vi "Principal.vi"() -> ()   [LabVIEW 2018]
panel:
  out "Time":string
  out "Date":string
  out "VIs ref":refnum<vi>[](array[refnum])
  in  "Reports":bool
  in  "Network":bool
  in  "Configuration":bool
  in  "Trends":bool
  in  "Overview":bool
  in  "Return 2":bool
  in  "Return":bool
  in  "Boton Tanque 4":bool
  out "Tank 4":dbl(slide)=80.0 scale=0.0..100.0 scale format="%#_g%%"
  out "Pressure 4":dbl=14.0 format="%#_g psi"
  out "Fuel Level 4":dbl=800.0 format="%#_g L"
  out "Temperature 4":dbl=60.0 format="%#_g °C"
  out "Percentage 4":dbl=80.0 format="%#_g %%"
  in  "Boton Tanque 3":bool
  out "Tank 3":dbl(slide)=60.0 scale=0.0..100.0 scale format="%#_g%%"
  out "Pressure 3":dbl=13.0 format="%#_g psi"
  out "Fuel Level 3":dbl=600.0 format="%#_g L"
  out "Temperature 3":dbl=45.0 format="%#_g °C"
  out "Percentage 3":dbl=60.0 format="%#_g %%"
  in  "Boton Tanque 2":bool
  out "Tank 2":dbl(slide)=40.0 scale=0.0..100.0 scale format="%#_g%%"
  out "Pressure 2":dbl=12.0 format="%#_g psi"
  out "Fuel Level 2":dbl=400.0 format="%#_g L"
  out "Temperature 2":dbl=30.0 format="%#_g °C"
  out "Percentage 2":dbl=40.0 format="%#_g %%"
  in  "Boton Tanque 1":bool
  out "Tank 1":dbl(slide)=20.0 scale=0.0..100.0 scale format="%#_g%%"
  out "Pressure":dbl=11.0 format="%#_g psi"
  out "Fuel Level":dbl=200.0 format="%#_g L"
  out "Temperature":dbl=15.0 format="%#_g °C"
  out "Percentage":dbl=20.0 format="%.0f %%"
  in  "stop":bool
  in  "SideTank4":bool
  in  "SideTank3":bool
  in  "SideTank2":bool
  in  "SideTank1":bool
  in  "Down Button":bool
  in  "Up Button":bool
  out "Multicolumn Listbox":i32(listbox)=5
  # "Fuel Tanks Gauging System - Tanks Courtyard \"Name\""
  # "View Tanks Details"
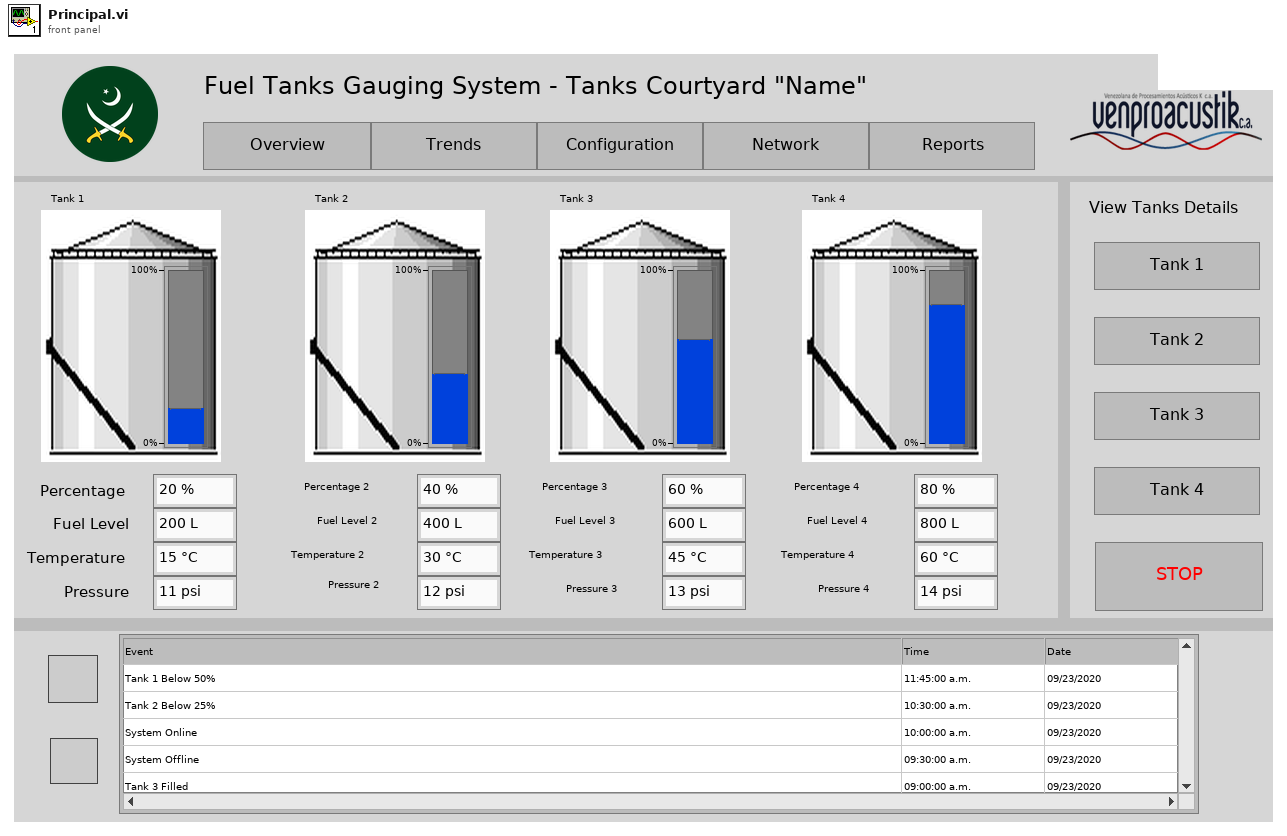
[diagram p1: front panel]
types:
  T1 = cluster{"Pressure":dbl, "Fuel Level":dbl, "Temperature":dbl, "Percentage":dbl}
  T2 = cluster{"Pressure 2":dbl, "Fuel Level 2":dbl, "Temperature 2":dbl, "Percentage 2":dbl}
  T3 = cluster{"Pressure 3":dbl, "Fuel Level 3":dbl, "Temperature 3":dbl, "Percentage 3":dbl}
  T4 = cluster{"Pressure 4":dbl, "Fuel Level 4":dbl, "Temperature 4":dbl, "Percentage 4":dbl}
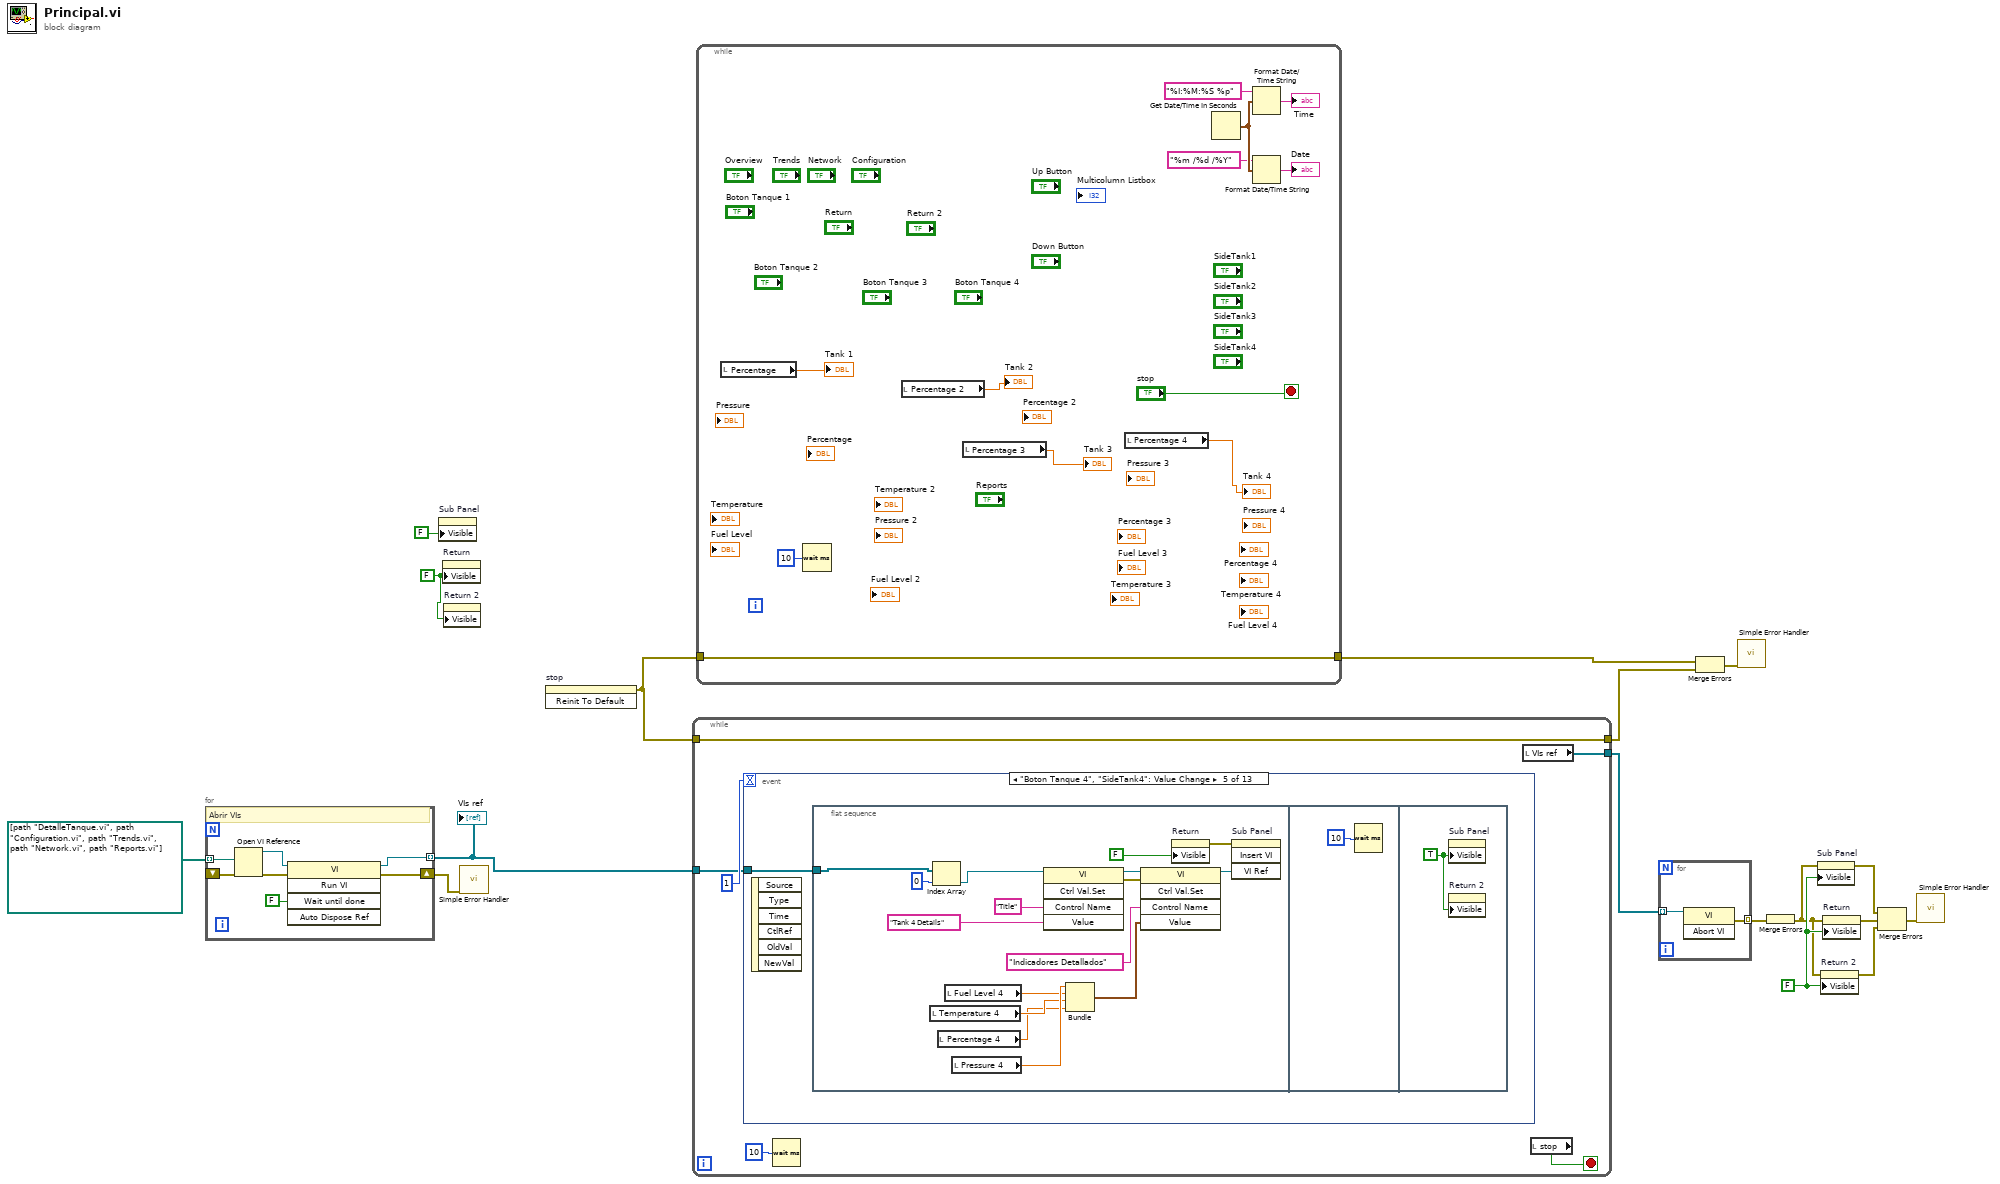
[diagram p0: block diagram]
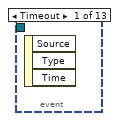
[diagram p2: hidden frame]
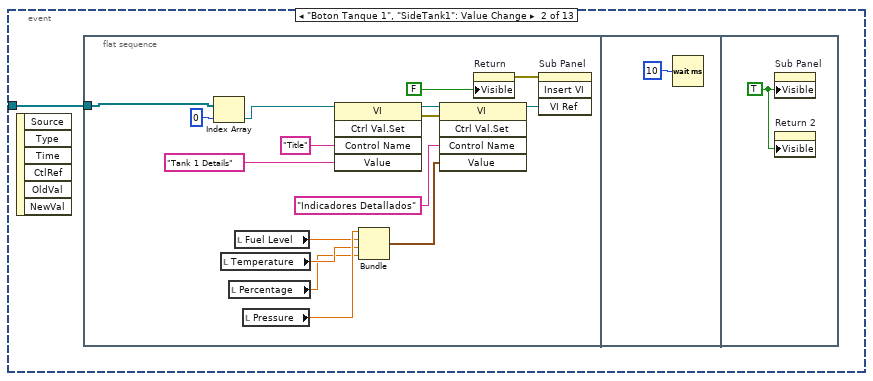
[diagram p3: hidden frame]
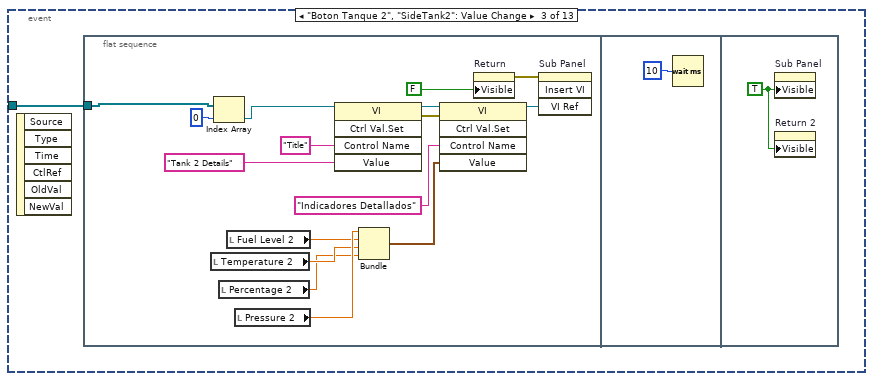
[diagram p4: hidden frame]
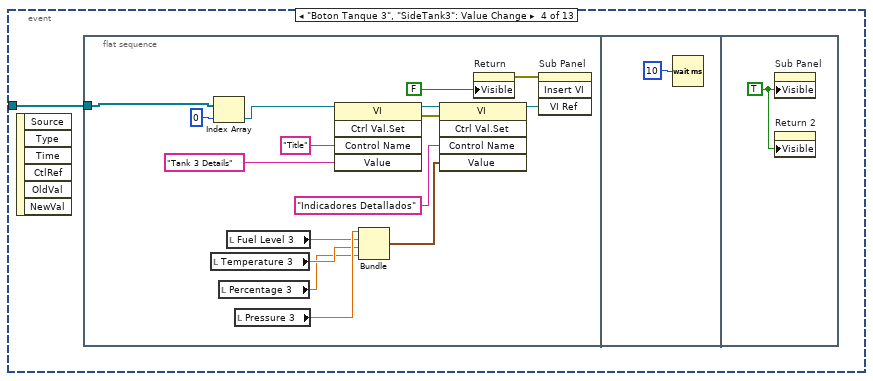
[diagram p5: hidden frame]
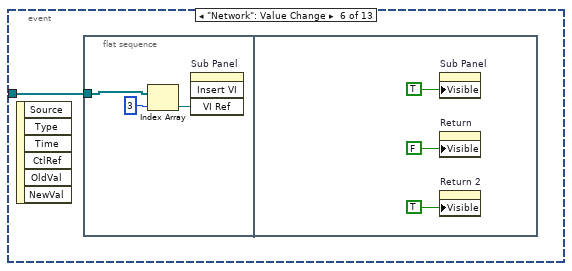
[diagram p6: hidden frame]
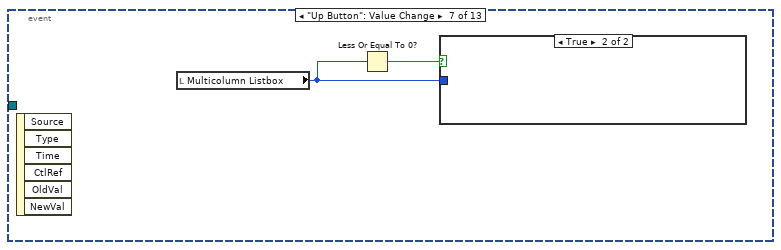
[diagram p7: hidden frame]
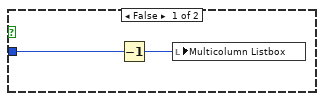
[diagram p8: hidden frame]
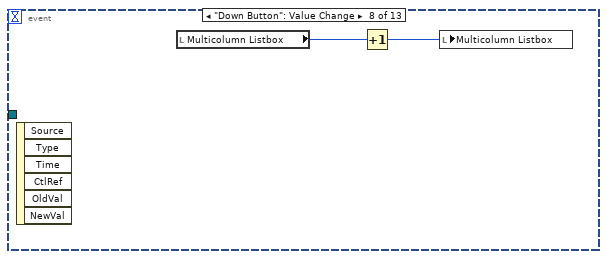
[diagram p9: hidden frame]
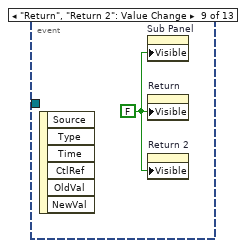
[diagram p10: hidden frame]
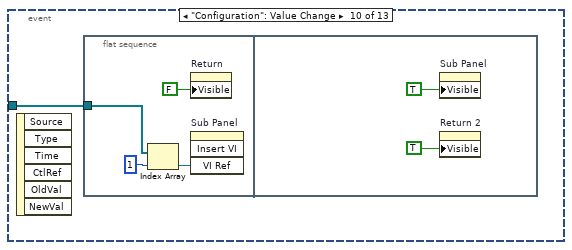
[diagram p11: hidden frame]
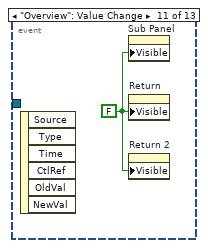
[diagram p12: hidden frame]
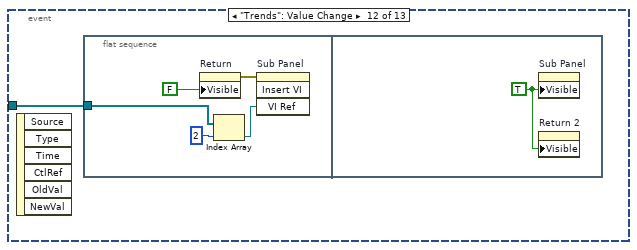
[diagram p13: hidden frame]
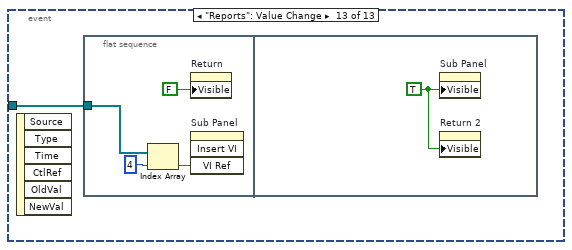
[diagram p14: hidden frame]
diagram:
  w7 = FALSE ("Visible")
  w8 = FALSE ("Visible")
  n1 = for {
    tunnel: path[] [path "DetalleTanque.vi", path "Configuration.vi", path "Trends.vi", path "Network.vi", path "Reports.vi"] -> [w24] mode=indexing
    shift-right: [w20] -> w12
    shift-left: _ -> [w19]
    tunnel: [w18] -> w1 mode=indexing
    # "Abrir VIs"
    n2 = Open VI Reference(vi path=w24, error in (no error)=w19) -> (vi reference=w22:refnum<vi>, error out=w21:errorcluster)  [unwired: 4 in]
    n3 = invoke class="VI" method="Run VI"(reference=w22, error in=w21, "Wait until done"=FALSE ("Wait Until Done")) -> (reference out=w18:refnum<vi>, error out=w20:errorcluster)  [unwired: 2 in, 3 out]
  }
  "VIs ref" <- w1
  n4 = property on="Sub Panel" class="SubPnl"("Visible"=FALSE) -> ()  [unwired: 2 in, 2 out]
  n5 = property on="Return" class="Bool"("Visible"=w8) -> ()  [unwired: 2 in, 2 out]
  n6 = property on="Return 2" class="Bool"("Visible"=w8) -> ()  [unwired: 2 in, 2 out]
  n7 = call <vilib>:"Simple Error Handler.vi"("error in (no error)"=w12) -> ()  [unwired: 4 in, 5 out]
  n8 = invoke on="stop" class="Bool (strict)" method="Reinit To Default"() -> (error out=w9:errorcluster)  [unwired: 3 in, 2 out]
  n9 = while {
    tunnel: w9 -> [w28]
    tunnel: [w28] -> w15
    tunnel: w1 -> [w27]
    tunnel: [w26] -> w11
    stop <- w29 stop-if-true
    n10 = event shown="[4] \"Boton Tanque 4\", \"SideTank4\": Value Change" {
      selector: _ -> [_ _ _ _ _ _ _ _ _ _ _ _ _]
      dyn-events: _ -> [_ _ _ _ _ _ _ _ _ _ _ _ _]
      timeout: 1 -> [_ _ _ _ _ _ _ _ _ _ _ _ _]
      tunnel: w27 -> [_ w31 w50 w69 w88 w107 _ _ _ w121 _ w129 w136]
      event Timeout {
        n11 = event-data() -> ()  [unwired: 1 in, 3 out]
      }
      event "Boton Tanque 1", "SideTank1": Value Change {
        n12 = event-data() -> ()  [unwired: 1 in, 6 out]
        n13 = flat-sequence {
          tunnel: w31 -> [w36]
          frame #0 {
            n14 = Index Array(array=w36, index=0) -> (element=w35:refnum<vi>)
            n15 = local read "Temperature"() -> (w41:dbl)
            n16 = local read "Percentage"() -> (w40:dbl)
            n17 = local read "Fuel Level"() -> (w42:dbl)
            n18 = local read "Pressure"() -> (w43:dbl)
            n19 = invoke class="VI" method="Ctrl Val.Set"(reference=w35, "Control Name"="Title", "Value"="Tank 1 Details" ("Control Name")) -> (reference out=w45:refnum<vi>, error out=w44:errorcluster)  [unwired: 2 in, 3 out]
            n20 = Bundle("Pressure"=w43, "Fuel Level"=w42, "Temperature"=w41, "Percentage"=w40) -> (w37:T1)  [unwired: 1 in]
            n21 = invoke class="VI" method="Ctrl Val.Set"(reference=w45, error in=w44, "Control Name"="Indicadores Detallados", "Value"=w37) -> (reference out=w38:refnum<vi>)  [unwired: 1 in, 4 out]
            n22 = property on="Return" class="Bool"("Visible"=FALSE) -> (error out=w32:errorcluster)  [unwired: 2 in, 1 out]
            n23 = invoke on="Sub Panel" class="SubPnl" method="Insert VI"(error in=w32, "VI Ref"=w38) -> ()  [unwired: 2 in, 4 out]
          }
          frame #1 {
            n24 = Wait (ms)(milliseconds to wait=u32 10) -> ()  [unwired: 1 out]
          }
          frame #2 {
            w49 = TRUE ("Visible")
            n25 = property on="Sub Panel" class="SubPnl"("Visible"=w49) -> ()  [unwired: 2 in, 2 out]
            n26 = property on="Return 2" class="Bool"("Visible"=w49) -> ()  [unwired: 2 in, 2 out]
          }
        }
      }
      event "Boton Tanque 2", "SideTank2": Value Change {
        n27 = event-data() -> ()  [unwired: 1 in, 6 out]
        n28 = flat-sequence {
          tunnel: w50 -> [w53]
          frame #0 {
            n29 = local read "Temperature 2"() -> (w60:dbl)
            n30 = Index Array(array=w53, index=0) -> (element=w54:refnum<vi>)
            n31 = local read "Percentage 2"() -> (w59:dbl)
            n32 = local read "Fuel Level 2"() -> (w61:dbl)
            n33 = local read "Pressure 2"() -> (w62:dbl)
            n34 = invoke class="VI" method="Ctrl Val.Set"(reference=w54, "Control Name"="Title", "Value"="Tank 2 Details" ("Control Name")) -> (reference out=w64:refnum<vi>, error out=w63:errorcluster)  [unwired: 2 in, 3 out]
            n35 = Bundle("Pressure 2"=w62, "Fuel Level 2"=w61, "Temperature 2"=w60, "Percentage 2"=w59) -> (w56:T2)  [unwired: 1 in]
            n36 = invoke class="VI" method="Ctrl Val.Set"(reference=w64, error in=w63, "Control Name"="Indicadores Detallados", "Value"=w56) -> (reference out=w57:refnum<vi>)  [unwired: 1 in, 4 out]
            n37 = property on="Return" class="Bool"("Visible"=FALSE) -> (error out=w51:errorcluster)  [unwired: 2 in, 1 out]
            n38 = invoke on="Sub Panel" class="SubPnl" method="Insert VI"(error in=w51, "VI Ref"=w57) -> ()  [unwired: 2 in, 4 out]
          }
          frame #1 {
            n39 = Wait (ms)(milliseconds to wait=u32 10) -> ()  [unwired: 1 out]
          }
          frame #2 {
            w68 = TRUE ("Visible")
            n40 = property on="Sub Panel" class="SubPnl"("Visible"=w68) -> ()  [unwired: 2 in, 2 out]
            n41 = property on="Return 2" class="Bool"("Visible"=w68) -> ()  [unwired: 2 in, 2 out]
          }
        }
      }
      event "Boton Tanque 3", "SideTank3": Value Change {
        n42 = event-data() -> ()  [unwired: 1 in, 6 out]
        n43 = flat-sequence {
          tunnel: w69 -> [w73]
          frame #0 {
            n44 = local read "Temperature 3"() -> (w79:dbl)
            n45 = Index Array(array=w73, index=0) -> (element=w72:refnum<vi>)
            n46 = local read "Percentage 3"() -> (w78:dbl)
            n47 = local read "Fuel Level 3"() -> (w80:dbl)
            n48 = local read "Pressure 3"() -> (w81:dbl)
            n49 = invoke class="VI" method="Ctrl Val.Set"(reference=w72, "Control Name"="Title", "Value"="Tank 3 Details" ("Control Name")) -> (reference out=w83:refnum<vi>, error out=w82:errorcluster)  [unwired: 2 in, 3 out]
            n50 = Bundle("Pressure 3"=w81, "Fuel Level 3"=w80, "Temperature 3"=w79, "Percentage 3"=w78) -> (w75:T3)  [unwired: 1 in]
            n51 = invoke class="VI" method="Ctrl Val.Set"(reference=w83, error in=w82, "Control Name"="Indicadores Detallados", "Value"=w75) -> (reference out=w76:refnum<vi>)  [unwired: 1 in, 4 out]
            n52 = property on="Return" class="Bool"("Visible"=FALSE) -> (error out=w71:errorcluster)  [unwired: 2 in, 1 out]
            n53 = invoke on="Sub Panel" class="SubPnl" method="Insert VI"(error in=w71, "VI Ref"=w76) -> ()  [unwired: 2 in, 4 out]
          }
          frame #1 {
            n54 = Wait (ms)(milliseconds to wait=u32 10) -> ()  [unwired: 1 out]
          }
          frame #2 {
            w87 = TRUE ("Visible")
            n55 = property on="Sub Panel" class="SubPnl"("Visible"=w87) -> ()  [unwired: 2 in, 2 out]
            n56 = property on="Return 2" class="Bool"("Visible"=w87) -> ()  [unwired: 2 in, 2 out]
          }
        }
      }
      event "Boton Tanque 4", "SideTank4": Value Change {
        n57 = event-data() -> ()  [unwired: 1 in, 6 out]
        n58 = flat-sequence {
          tunnel: w88 -> [w92]
          frame #0 {
            n59 = local read "Temperature 4"() -> (w98:dbl)
            n60 = Index Array(array=w92, index=0) -> (element=w91:refnum<vi>)
            n61 = local read "Percentage 4"() -> (w97:dbl)
            n62 = local read "Fuel Level 4"() -> (w99:dbl)
            n63 = local read "Pressure 4"() -> (w100:dbl)
            n64 = invoke class="VI" method="Ctrl Val.Set"(reference=w91, "Control Name"="Title", "Value"="Tank 4 Details" ("Control Name")) -> (reference out=w102:refnum<vi>, error out=w101:errorcluster)  [unwired: 2 in, 3 out]
            n65 = Bundle("Pressure 4"=w100, "Fuel Level 4"=w99, "Temperature 4"=w98, "Percentage 4"=w97) -> (w94:T4)  [unwired: 1 in]
            n66 = invoke class="VI" method="Ctrl Val.Set"(reference=w102, error in=w101, "Control Name"="Indicadores Detallados", "Value"=w94) -> (reference out=w95:refnum<vi>)  [unwired: 1 in, 4 out]
            n67 = property on="Return" class="Bool"("Visible"=FALSE) -> (error out=w89:errorcluster)  [unwired: 2 in, 1 out]
            n68 = invoke on="Sub Panel" class="SubPnl" method="Insert VI"(error in=w89, "VI Ref"=w95) -> ()  [unwired: 2 in, 4 out]
          }
          frame #1 {
            n69 = Wait (ms)(milliseconds to wait=u32 10) -> ()  [unwired: 1 out]
          }
          frame #2 {
            w106 = TRUE ("Visible")
            n70 = property on="Sub Panel" class="SubPnl"("Visible"=w106) -> ()  [unwired: 2 in, 2 out]
            n71 = property on="Return 2" class="Bool"("Visible"=w106) -> ()  [unwired: 2 in, 2 out]
          }
        }
      }
      event "Network": Value Change {
        n72 = event-data() -> ()  [unwired: 1 in, 6 out]
        n73 = flat-sequence {
          tunnel: w107 -> [w108]
          frame #0 {
            n74 = Index Array(array=w108, index=3) -> (element=w109:refnum<vi>)
            n75 = invoke on="Sub Panel" class="SubPnl" method="Insert VI"("VI Ref"=w109) -> ()  [unwired: 3 in, 4 out]
          }
          frame #1 {
            n76 = property on="Sub Panel" class="SubPnl"("Visible"=TRUE) -> ()  [unwired: 2 in, 2 out]
            n77 = property on="Return" class="Bool"("Visible"=FALSE) -> ()  [unwired: 2 in, 2 out]
            n78 = property on="Return 2" class="Bool"("Visible"=TRUE) -> ()  [unwired: 2 in, 2 out]
          }
        }
      }
      event "Up Button": Value Change {
        n79 = event-data() -> ()  [unwired: 1 in, 6 out]
        n80 = local read "Multicolumn Listbox"() -> (w114:i32)
        n81 = Less Or Equal To 0?(x=w114) -> (x <= 0?=w115:bool)
        n82 = case shown="True" w115 {
          tunnel: w114 -> [w116 _]
          frame False {
            n83 = Decrement(x=w116) -> (x-1=w117:i32)
            n84 = local write "Multicolumn Listbox"(w117) -> ()
          }
          frame True {
          }
        }
      }
      event "Down Button": Value Change {
        n85 = event-data() -> ()  [unwired: 1 in, 6 out]
        n86 = local read "Multicolumn Listbox"() -> (w119:i32)
        n87 = Increment(x=w119) -> (x+1=w118:i32)
        n88 = local write "Multicolumn Listbox"(w118) -> ()
      }
      event "Return", "Return 2": Value Change {
        w120 = FALSE ("Visible")
        n89 = event-data() -> ()  [unwired: 1 in, 6 out]
        n90 = property on="Sub Panel" class="SubPnl"("Visible"=w120) -> ()  [unwired: 2 in, 2 out]
        n91 = property on="Return" class="Bool"("Visible"=w120) -> ()  [unwired: 2 in, 2 out]
        n92 = property on="Return 2" class="Bool"("Visible"=w120) -> ()  [unwired: 2 in, 2 out]
      }
      event "Configuration": Value Change {
        n93 = event-data() -> ()  [unwired: 1 in, 6 out]
        n94 = flat-sequence {
          tunnel: w121 -> [w124]
          frame #0 {
            n95 = Index Array(array=w124, index=1) -> (element=w123:refnum<vi>)
            n96 = property on="Return" class="Bool"("Visible"=FALSE) -> ()  [unwired: 2 in, 2 out]
            n97 = invoke on="Sub Panel" class="SubPnl" method="Insert VI"("VI Ref"=w123) -> ()  [unwired: 3 in, 4 out]
          }
          frame #1 {
            n98 = property on="Sub Panel" class="SubPnl"("Visible"=TRUE) -> ()  [unwired: 2 in, 2 out]
            n99 = property on="Return 2" class="Bool"("Visible"=TRUE) -> ()  [unwired: 2 in, 2 out]
          }
        }
      }
      event "Overview": Value Change {
        w128 = FALSE ("Visible")
        n100 = event-data() -> ()  [unwired: 1 in, 6 out]
        n101 = property on="Sub Panel" class="SubPnl"("Visible"=w128) -> ()  [unwired: 2 in, 2 out]
        n102 = property on="Return" class="Bool"("Visible"=w128) -> ()  [unwired: 2 in, 2 out]
        n103 = property on="Return 2" class="Bool"("Visible"=w128) -> ()  [unwired: 2 in, 2 out]
      }
      event "Trends": Value Change {
        n104 = event-data() -> ()  [unwired: 1 in, 6 out]
        n105 = flat-sequence {
          tunnel: w129 -> [w132]
          frame #0 {
            n106 = property on="Return" class="Bool"("Visible"=FALSE) -> (error out=w130:errorcluster)  [unwired: 2 in, 1 out]
            n107 = Index Array(array=w132, index=2) -> (element=w133:refnum<vi>)
            n108 = invoke on="Sub Panel" class="SubPnl" method="Insert VI"(error in=w130, "VI Ref"=w133) -> ()  [unwired: 2 in, 4 out]
          }
          frame #1 {
            w135 = TRUE ("Visible")
            n109 = property on="Sub Panel" class="SubPnl"("Visible"=w135) -> ()  [unwired: 2 in, 2 out]
            n110 = property on="Return 2" class="Bool"("Visible"=w135) -> ()  [unwired: 2 in, 2 out]
          }
        }
      }
      event "Reports": Value Change {
        n111 = event-data() -> ()  [unwired: 1 in, 6 out]
        n112 = flat-sequence {
          tunnel: w136 -> [w139]
          frame #0 {
            n113 = Index Array(array=w139, index=4) -> (element=w138:refnum<vi>)
            n114 = property on="Return" class="Bool"("Visible"=FALSE) -> ()  [unwired: 2 in, 2 out]
            n115 = invoke on="Sub Panel" class="SubPnl" method="Insert VI"("VI Ref"=w138) -> ()  [unwired: 3 in, 4 out]
          }
          frame #1 {
            w141 = TRUE ("Visible")
            n116 = property on="Sub Panel" class="SubPnl"("Visible"=w141) -> ()  [unwired: 2 in, 2 out]
            n117 = property on="Return 2" class="Bool"("Visible"=w141) -> ()  [unwired: 2 in, 2 out]
          }
        }
      }
    }
    n118 = Wait (ms)(milliseconds to wait=u32 10) -> ()  [unwired: 1 out]
    n119 = local read "VIs ref"() -> (w26:refnum<vi>[])
    n120 = local read "stop"() -> (w29:bool)
  }
  n121 = while {
    tunnel: [w147] -> w16
    tunnel: w9 -> [w147]
    stop <- "stop" stop-if-true
    n122 = local read "Percentage"() -> (→"Tank 1":dbl)
    n123 = Wait (ms)(milliseconds to wait=u32 10) -> ()  [unwired: 1 out]
    n124 = local read "Percentage 2"() -> (→"Tank 2":dbl)
    n125 = local read "Percentage 3"() -> (→"Tank 3":dbl)
    n126 = local read "Percentage 4"() -> (→"Tank 4":dbl)
    n127 = Get Date/Time In Seconds() -> (seconds since 1Jan1904=w144:timestamp)
    n128 = Format Date/Time String(time format string (%c)="%I:%M:%S %p", seconds (now)=w144) -> (date/time string=→"Time":string)  [unwired: 1 in]
    n129 = Format Date/Time String(time format string (%c)="%m /%d /%Y", seconds (now)=w144) -> (date/time string=→"Date":string)  [unwired: 1 in]
  }
  n130 = for {
    tunnel: w11 -> [w155] mode=indexing
    tunnel: [w154] -> w10 mode=indexing
    n131 = invoke class="VI" method="Abort VI"(reference=w155) -> (error out=w154:errorcluster)  [unwired: 2 in, 2 out]
  }
  n132 = Merge Errors(w16, w15) -> (w14:errorcluster)
  n133 = call <vilib>:"Simple Error Handler.vi"("error in (no error)"=w14) -> ()  [unwired: 4 in, 5 out]
  n134 = Merge Errors(w10) -> (w6:errorcluster)
  n135 = property on="Sub Panel" class="SubPnl"(error in=w6, "Visible"=w7) -> (error out=w4:errorcluster)  [unwired: 1 in, 1 out]
  n136 = property on="Return 2" class="Bool"(error in=w6, "Visible"=w7) -> (error out=w2:errorcluster)  [unwired: 1 in, 1 out]
  n137 = property on="Return" class="Bool"(error in=w6, "Visible"=w7) -> (error out=w3:errorcluster)  [unwired: 1 in, 1 out]
  n138 = Merge Errors(w4, w3, w2) -> (w5:errorcluster)
  n139 = call <vilib>:"Simple Error Handler.vi"("error in (no error)"=w5) -> ()  [unwired: 4 in, 5 out]
